vi "make_recording_h5_files.vi"(10 "write/append size":i32=1000, 11 "Path":path) -> (0 "error out":errorcluster, 2 "dataset cluster":T1, 3 "ref out":T2 format="%.0x")   [LabVIEW 2015]
uses:
  <vilib>/addons/h5labview2/base/hid_t.ctl
  <vilib>/addons/h5labview2/file/H5Fmode.ctl
  <vilib>/addons/h5labview2/base/lib_path.vi
  <vilib>/addons/h5labview2/base/H5Equery.vi
  <vilib>/addons/h5labview2/attrib/H5Awrite.llb/H5Awrite.xnode
  <vilib>/addons/h5labview2/file/H5F.lvlib
  <vilib>/addons/h5labview2/group/H5G.lvlib
  <vilib>/addons/h5labview2/dataset/H5D.lvlib
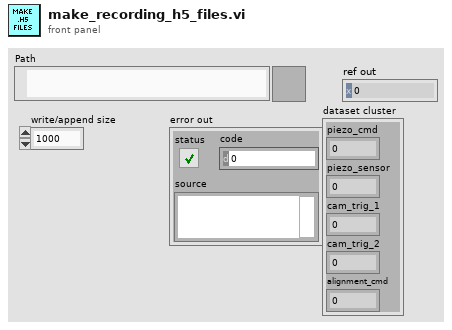
[diagram p1: front panel]
types:
  T1 = cluster{"piezo_cmd":i32, "piezo_sensor":i32, "cam_trig_1":i32, "cam_trig_2":i32, "alignment_cmd":i32}
  T2 = typedef "hid_t.ctl" = i32
  T3 = typedef "H5F.lvlib/H5Fmode.ctl" = enum16{"read-only", "read-write", "overwrite", "create new", "open or create"}
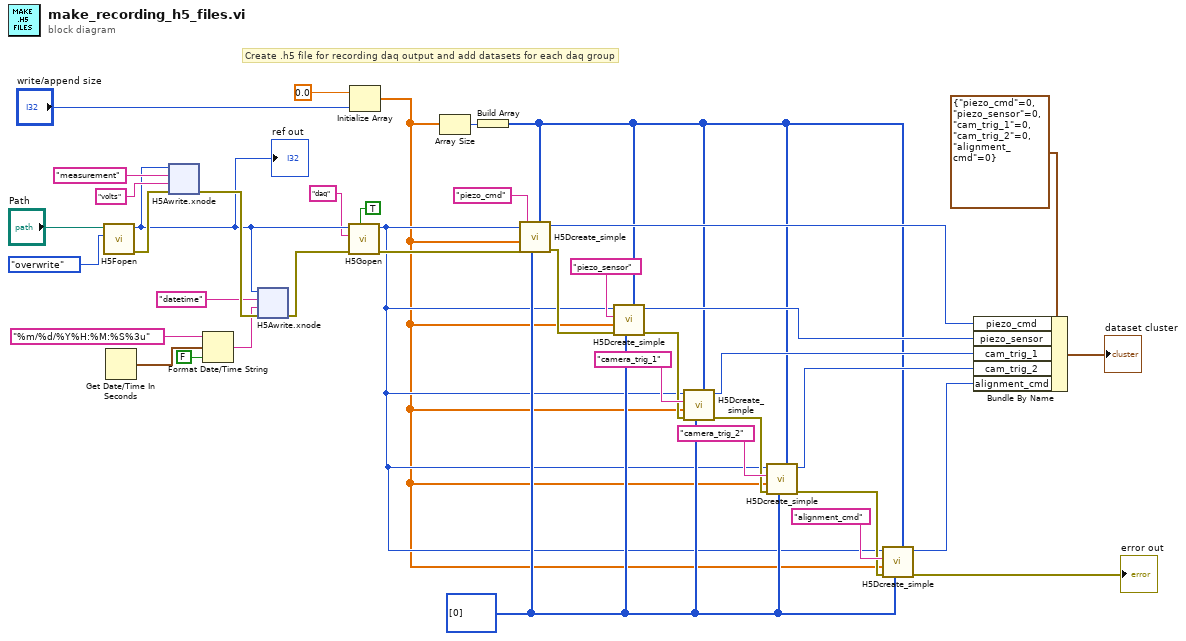
[diagram p0: block diagram]
diagram:
  w7 = i32[] [0] ("initial size")
  # "Create .h5 file for recording daq output and add datasets for each daq group"
  n1 = call <vilib>:"H5Fopen.vi"("mode (read-only)"=H5Fmode."overwrite" ("mode"), "path"="Path") -> ("error out"=w38:errorcluster, "ref out"=w35:T2)  [unwired: 8 in]
  "ref out" <- w35
  n2 = Get Date/Time In Seconds() -> (seconds since 1Jan1904=w29:timestamp)
  n3 = xnode "H5Awrite.xnode"("error in (no error)"=w38, "data"="volts" ("name"), "attrib name"="measurement" ("name"), "ref in"=w35) -> ("error out"=w39:errorcluster)  [unwired: 3 in, 2 out]
  n4 = Format Date/Time String(time format string (%c)="%m/%d/%Y%H:%M:%S%3u", seconds (now)=w29, UTC format=FALSE ("want seconds? (F)")) -> (date/time string=w27:string)
  n5 = xnode "H5Awrite.xnode"("error in (no error)"=w39, "data"=w27, "attrib name"="datetime" ("name"), "ref in"=w35) -> ("error out"=w40:errorcluster)  [unwired: 3 in, 2 out]
  n6 = call <vilib>:"H5Gopen.vi"("create? (F)"=TRUE, "error in (no error)"=w40, "name"="daq", "ref in"=w35) -> ("error out"=w32:errorcluster, "group out"=w3:T2)  [unwired: 6 in]
  n7 = Initialize Array(0.0 ("element"), "write/append size") -> (w1:dbl[])
  n8 = Array Size(array=w1) -> (size(s)=w19:i32)
  n9 = Build Array(w19) -> (w2:i32[])
  n10 = call <vilib>:"H5Dcreate_simple.vi"("chunk size"=w2, "initial size"=w7, "error in (no error)"=w32, "type in"=w1, "name"="piezo_cmd", "ref in"=w3) -> ("error out"=w34:errorcluster, "dset out"=w13:T2)  [unwired: 4 in]
  n11 = call <vilib>:"H5Dcreate_simple.vi"("chunk size"=w2, "initial size"=w7, "error in (no error)"=w34, "type in"=w1, "name"="piezo_sensor", "ref in"=w3) -> ("error out"=w17:errorcluster, "dset out"=w12:T2)  [unwired: 4 in]
  n12 = call <vilib>:"H5Dcreate_simple.vi"("chunk size"=w2, "initial size"=w7, "error in (no error)"=w17, "type in"=w1, "name"="camera_trig_1", "ref in"=w3) -> ("error out"=w15:errorcluster, "dset out"=w11:T2)  [unwired: 4 in]
  n13 = call <vilib>:"H5Dcreate_simple.vi"("chunk size"=w2, "initial size"=w7, "error in (no error)"=w15, "type in"=w1, "name"="camera_trig_2", "ref in"=w3) -> ("error out"=w6:errorcluster, "dset out"=w10:T2)  [unwired: 4 in]
  n14 = call <vilib>:"H5Dcreate_simple.vi"("chunk size"=w2, "initial size"=w7, "error in (no error)"=w6, "type in"=w1, "name"="alignment_cmd", "ref in"=w3) -> ("error out"=→"error out":errorcluster, "dset out"=w4:T2)  [unwired: 4 in]
  n15 = Bundle By Name(cluster=T1 {"piezo_cmd"=0, "piezo_sensor"=0, "cam_trig_1"=0, "cam_trig_2"=0, "alignment_cmd"=0}, "piezo_cmd"=w13, "piezo_sensor"=w12, "cam_trig_1"=w11, "cam_trig_2"=w10, "alignment_cmd"=w4) -> (→"dataset cluster":T1)
